vi "Parse .hex File.vi"(0 "file path":path=path "C:/Users/CR Filipe/Documents/BitBucket/Device.Wear.Basestation/Firmware/Master/Debug/Master.hex", 11 "error in":errorcluster) -> (8 ".hex lines":T1(array[cluster]), 15 "error out":errorcluster)   [LabVIEW 2010]
panel:
  in  ".hex line":T2
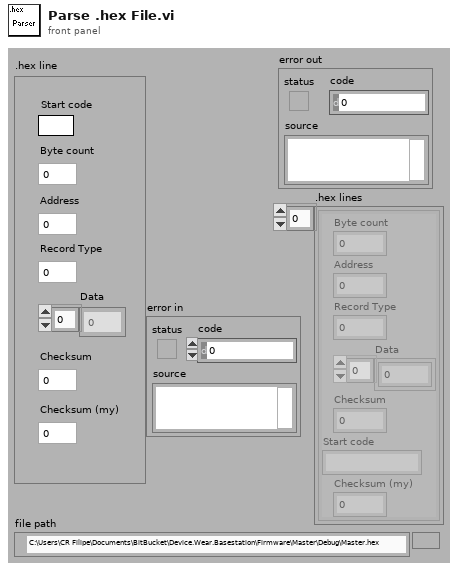
[diagram p1: front panel]
types:
  T1 = cluster{"Byte count":u8, "Address":u16, "Record Type":u8, "Data":u8[], "Checksum":u8, "Start code":string, "Checksum (my)":u8}[]
  T2 = cluster{"Byte count":u8, "Address":u16, "Record Type":u8, "Data":u8[], "Checksum":u8, "Start code":string, "Checksum (my)":u8}
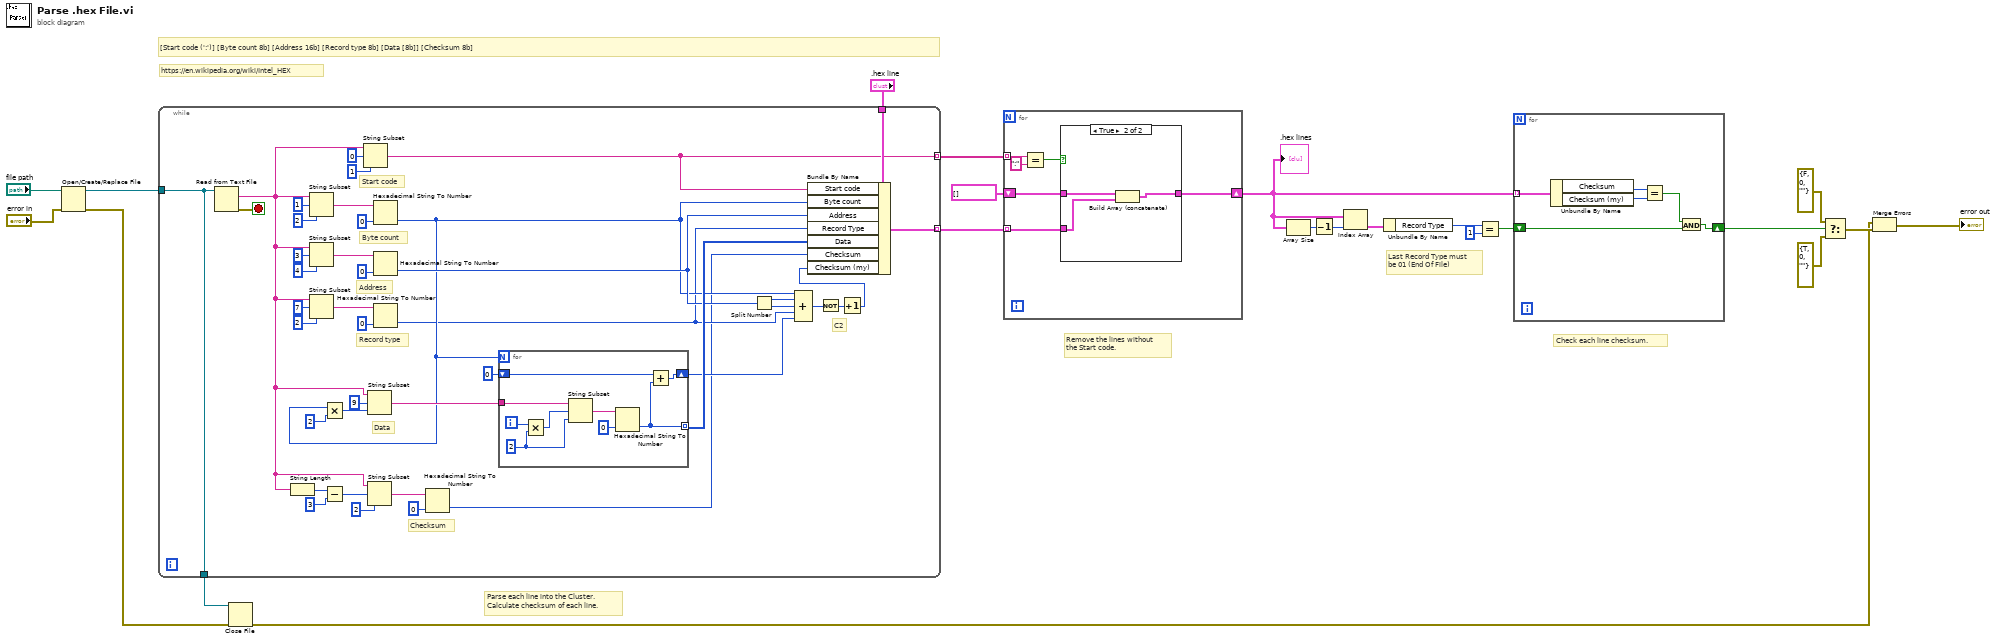
[diagram p0: block diagram]
diagram:
  # "Parse each line into the Cluster.\nCalculate checksum of each line."
  # "Remove the lines without\nthe Start code."
  # "Check each line checksum."
  # "https://en.wikipedia.org/wiki/Intel_HEX"
  # "Last Record Type must\nbe 01 (End Of File)"
  # "[Start code (':')] [Byte count 8b] [Address 16b] [Record type 8b] [Data [8b]] [Checksum 8b]"
  n1 = Open/Create/Replace File(file path (use dialog)="file path", error in="error in") -> (refnum out=w21:refnum<file>, error out=w6:errorcluster)  [unwired: 4 in, 1 out]
  n2 = while {
    tunnel: w21 -> [w23]
    tunnel: ".hex line" -> [w38]
    tunnel: [w36] -> w17 mode=indexing
    tunnel: [w28] -> w19 mode=indexing
    tunnel: [w23] -> w7
    stop <- w64 stop-if-true
    # "C2"
    # "Data"
    # "Checksum"
    # "Record type"
    # "Address"
    # "Byte count"
    # "Start code"
    n3 = Read from Text File(file (use dialog)=w23) -> (text=w42:string, error out=w64:errorcluster)  [unwired: 3 in, 2 out]
    n4 = String Length(string=w42) -> (length=w48:i32)
    n5 = String Subset(string=w42, offset (0)=1, length (rest)=2 ("length (rest)")) -> (substring=w61:string)
    n6 = String Subset(string=w42, offset (0)=3, length (rest)=4 ("length (rest)")) -> (substring=w58:string)
    n7 = String Subset(string=w42, offset (0)=7, length (rest)=2 ("length (rest)")) -> (substring=w52:string)
    n8 = Subtract(x=w48, y=3) -> (x-y=w46:i32)
    n9 = String Subset(string=w42, offset (0)=0, length (rest)=1 ("length (rest)")) -> (substring=w28:string)
    n10 = String Subset(string=w42, offset (0)=w46, length (rest)=2 ("length (rest)")) -> (substring=w44:string)
    n11 = Hexadecimal String To Number(string=w61, default (0uL)=u8 0 ("default (0 U32)")) -> (number=w32:u8)  [unwired: 1 in, 1 out]
    n12 = Multiply(x=w32, y=2) -> (x*y=w41:i32)
    n13 = String Subset(string=w42, offset (0)=9 ("length (rest)"), length (rest)=w41) -> (substring=w39:string)
    n14 = Hexadecimal String To Number(string=w58, default (0uL)=u16 0 ("default (0 U32)")) -> (number=w35:u16)  [unwired: 1 in, 1 out]
    n15 = Hexadecimal String To Number(string=w52, default (0uL)=u8 0 ("default (0 U32)")) -> (number=w31:u8)  [unwired: 1 in, 1 out]
    n16 = Hexadecimal String To Number(string=w44, default (0uL)=u8 0 ("default (0 U32)")) -> (number=w27:u8)  [unwired: 1 in, 1 out]
    n17 = for {
      N: w32 -> [_]
      tunnel: w39 -> [w73]
      tunnel: [w67] -> w37 mode=indexing
      shift-right: [w65] -> w29
      shift-left: u8 0 ("x") -> [w66]
      i -> [w72]
      w70 = 2 ("y")
      n18 = Multiply(x=w72, y=w70) -> (x*y=w71:i32)
      n19 = String Subset(string=w73, offset (0)=w71, length (rest)=w70) -> (substring=w68:string)
      n20 = Hexadecimal String To Number(string=w68, default (0uL)=u8 0 ("default (0 U32)")) -> (number=w67:u8)  [unwired: 1 in, 1 out]
      n21 = Add(x=w66, y=w67) -> (x+y=w65:u8)
    }
    n22 = Split Number(x=w35) -> (hi(x)=w34:u8, lo(x)=w33:u8)
    n23 = Compound Arithmetic op=ADD(w32, w34, w33, w31, w29) -> (w25:u8)
    n24 = Not(x=w25) -> (.not. x?=w26:u8)
    n25 = Increment(x=w26) -> (x+1=w24:u8)
    n26 = Bundle By Name(cluster=w38, "Start code"=w28, "Byte count"=w32, "Address"=w35, "Record Type"=w31, "Data"=w37, "Checksum"=w27, "Checksum (my)"=w24) -> (w36:T2)
  }
  n27 = Close File(refnum=w7, error in=w6) -> (error out=w3:errorcluster)  [unwired: 1 out]
  n28 = for {
    tunnel: w17 -> [w79] mode=indexing
    shift-right: [w77] -> w12
    shift-left: T1 [] -> [w78]
    tunnel: w19 -> [w76] mode=indexing
    n29 = Equal?(x=w76, y=":") -> (x = y?=w74:bool)
    n30 = case shown="True" w74 {
      tunnel: w79 -> [_ w81]
      tunnel: w78 -> [w80 w83]
      tunnel: [w80 w82] -> w77
      frame False {
      }
      frame True {
        n31 = Build Array (concatenate)(w83, w81) -> (w82:T1)
      }
    }
  }
  ".hex lines" <- w12
  n32 = Array Size(array=w12) -> (size(s)=w18:i32)
  n33 = Decrement(x=w18) -> (x-1=w16:i32)
  n34 = Index Array(array=w12, index=w16) -> (element=w15:T2)
  n35 = Unbundle By Name(w15) -> ("Record Type"=w14:u8)
  n36 = Equal?(x=w14, y=u8 1) -> (x = y?=w10:bool)
  n37 = for {
    tunnel: w12 -> [w89] mode=indexing
    shift-right: [w86] -> w9
    shift-left: w10 -> [w85]
    n38 = Unbundle By Name(w89) -> ("Checksum"=w87:u8, "Checksum (my)"=w88:u8)
    n39 = Equal?(x=w87, y=w88) -> (x = y?=w84:bool)
    n40 = And(x=w84, y=w85) -> (x .and. y?=w86:bool)
  }
  n41 = Select(t=errorcluster {"status"=FALSE, "code"=0, "source"=""} ("error in (no error)"), s=w9, f=errorcluster {"status"=TRUE, "code"=0, "source"=""} ("error in (no error)")) -> (s? t:f=w4:errorcluster)
  n42 = Merge Errors(w3, w4) -> (→"error out":errorcluster)
